vi "L0_SUM_NOISE_TEST.vi"(7 "Serial Number":string="SN_026", 8 "error in (no error)":errorcluster, 11 "Instrument VISA in":T1={"AWG VISA"="AgilentGenerator1", "Oscilloscope  VISA "="AgilentOsciloscope", "Integration Board IP"="172.16.17.47", "connection ID"=refnum, "report out"=refnum, "report file path"=path "C:/Users/omartinez/Desktop/L0nL1_Results"}) -> (0 "error out":errorcluster, 3 "Instrument VISA out":T1={"AWG VISA"="AgilentGenerator1", "Oscilloscope  VISA "="AgilentOsciloscope", "Integration Board IP"="172.16.7.43", "connection ID"=refnum, "report out"=refnum, "report file path"=path "C:/Documents and Settings/CTA_LAB01/Desktop/L0_Asic/L0 Asic Test Data"})   [LabVIEW 2012]
uses:
  <vilib>/Utility/NIReport.llb/NI_report.lvclass
  <vilib>/Utility/NIReport.llb/HTML/NI_HTML.lvclass
  <instrlib>/Agilent 8000 Series/Public/Configure/Configure Math (Binary Operation).vi
  L0&L1/L0_BOARD_TESTs/trunk/Sum_Abrilader/L0_Sum_Adder Folder/C/Program Files/National Instruments/LabVIEW 2012/instr.lib/Agilent 8000 Series/Public/Data/Low Level/Fetch Measurement (More).vi
  <instrlib>/Agilent 8000 Series/Agilent 8000 Series.lvlib
panel:
  in  "Input Voltage":dbl=0.05
  in  "Amp Scaler":dbl=100.0
  in  "Ib_clipVb":u32=63
  in  "Clip_sel_b":u32=1
  in  "Att gain":u32
  in  "Delay value":u16
  in  "Gen Active":bool
  in  "Sum/Maj":bool
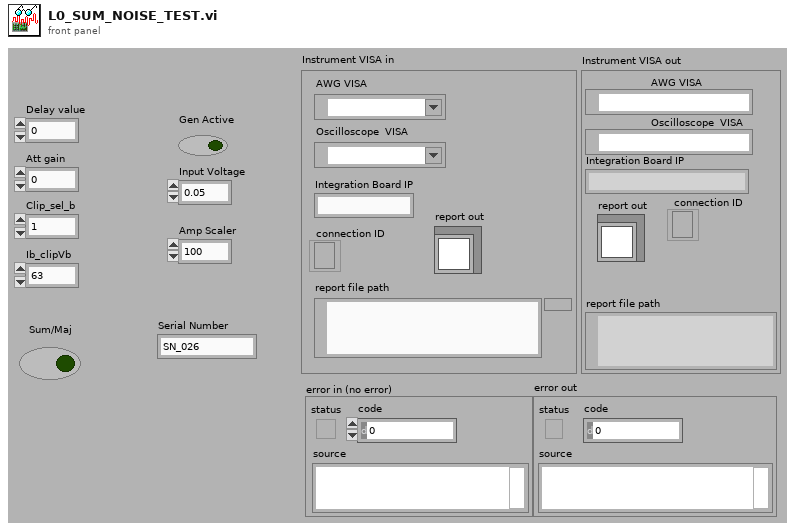
[diagram p1: front panel]
types:
  T1 = cluster{"AWG VISA":refnum<visa-resource-name>, "Oscilloscope  VISA ":refnum<visa-resource-name>, "Integration Board IP":string, "connection ID":refnum<k5>, "report out":refnum<class "NI_report.lvclass">, "report file path":path}
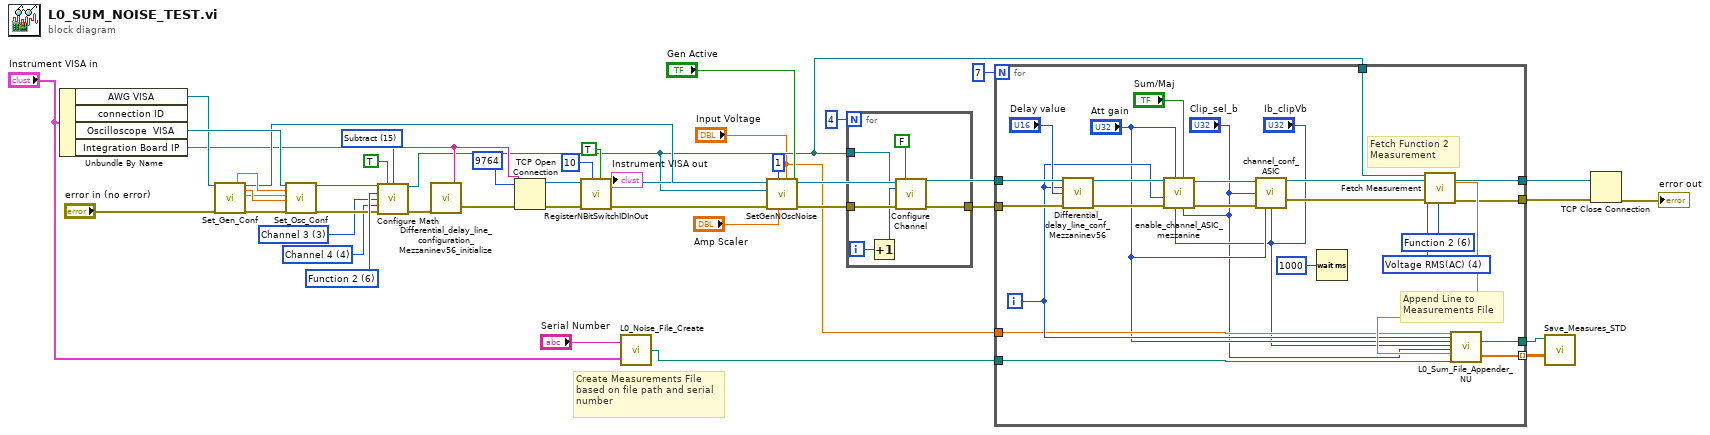
[diagram p0: block diagram]
diagram:
  w20 = u16 6 items=["Function 1"=5, "Function 2"=6, "Function 3"=7, "Function 4"=8] ("Math Channel (5: Function 1)")
  w21 = u16 15 items=["Add"=12, "Divide"=13, "Multiply"=14, "Subtract"=15, "Common Mode"=16, "Versus"=17] ("Math Operation (12: Add)")
  w15 = 3 items=["Channel 1"=1, "Channel 2"=2, "Channel 3"=3, "Channel 4"=4] ("Channel (1: Channel 1)")
  w16 = 4 items=["Channel 1"=1, "Channel 2"=2, "Channel 3"=3, "Channel 4"=4] ("Channel (1: Channel 1)")
  # "Create Measurements File\nbased on file path and serial\nnumber"
  n1 = Unbundle By Name("Instrument VISA in") -> ("AWG VISA"=w38:refnum<visa-resource-name>, "Oscilloscope  VISA"=w39:refnum<visa-resource-name>, "Integration Board IP"=w23:string)  [unwired: 1 out]
  n2 = call "Set_Gen_Conf.vi"("AWG VISA"=w38, "error in (no error)"="error in (no error)") -> ("Amplitude 1 OUT"=w36:dbl, "VISA resource name out"=w29:refnum<visa-resource-name>, "Pulse Width in seconds 1 OUT"=w35:dbl, "Trigger Level 1"=w34:dbl, "error out"=w40:errorcluster)  [unwired: 10 in, 3 out]
  n3 = call "Set_Osc_Conf.vi"("VISA resource name"=w39, "Amplitude IN"=w36, "Trigger Level IN"=w34, "Pulse Width in seconds IN"=w35, "error in (no error)"=w40) -> ("VISA resource name out"=w19:refnum<visa-resource-name>, "error out"=w18:errorcluster)  [unwired: 13 in]
  n4 = call-poly <instrlib>:"Configure Math.vi"("VISA resource name"=w19, "Enable Math Channel (T:Enable)"=TRUE, "Math Operation (12: Add)"=w21, "Math Channel (5: Function 1)"=w20, "Math Operand (1: Channel 1)"=w15, "Math Operand (2: Channel 2)"=w16, "error in (no error)"=w18) -> ("VISA resource name out"=w7:refnum<visa-resource-name>, "error out"=w17:errorcluster)  [unwired: 7 in]
  n5 = call "Differential_delay_line_configuration_Mezzaninev56_initialize.vi"("error in (no error)"=w17, "address"=w23) -> ("error out 2"=w33:errorcluster)
  n6 = TCP Open Connection(address=w23, remote port or service name=9764, error in (no error)=w33) -> (connection ID=w27:refnum<k5>, error out=w32:errorcluster)  [unwired: 2 in]
  n7 = call "RegisterNBitSwitchIDInOut.vi"("Switch Bit"=TRUE, "N Bit"=10, "error in (no error)"=w32, "connection ID"=w27) -> ("error out"=w28:errorcluster, "connection ID out"=w26:refnum<k5>)  [unwired: 5 in]
  n8 = call "L0_Noise_File_Create.vi"("input cluster"="Instrument VISA in", "Serial Number"="Serial Number") -> ("appended path"=w4:path)
  n9 = call "SetGenNOscNoise.vi"("Enable Output"="Gen Active", "Input Voltage"="Input Voltage", "Amp Scaler"="Amp Scaler", "NChannels"=1, "error in (no error)"=w28, "VISA resource name"=w7, "AWG VISA"=w29) -> ("error out 2"=w12:errorcluster)  [unwired: 4 in]
  n10 = for {
    N: 4 -> [_]
    tunnel: w12 -> [w48]
    tunnel: [w47] -> w11
    tunnel: w7 -> [w45]
    i -> [w46]
    n11 = Increment(x=w46) -> (x+1=w43:i32)
    n12 = call <instrlib>:"Configure Channel.vi"("VISA resource name"=w45, "Enable Channel (Enable)"=FALSE, "Channel (1: Channel 1)"=w43, "error in (no error)"=w48) -> ("error out"=w47:errorcluster)  [unwired: 10 in, 1 out]
  }
  n13 = for {
    N: 7 -> [_]
    tunnel: [w58] -> w31
    tunnel: [w72] -> w30
    tunnel: w26 -> [w71]
    tunnel: w11 -> [w63]
    tunnel: w7 -> [w57]
    tunnel: w4 -> [w56]
    tunnel: "Input Voltage" -> [w54]
    tunnel: [w50] -> w2
    tunnel: [w49] -> w1 mode=indexing
    i -> [w55]
    w60 = 4 items=["Rise Time", "Fall Time", "Frequency", "Period", "Voltage RMS(AC)", "Voltage RMS(DC)", "Voltage RMS (AC,cycle)", "Voltage RMS (DC,cycle)", "Voltage Max", "Voltage Min", "Voltage Middle", "Voltage Vpp", "Voltage High", "Voltage Low", "Voltage Average", "Voltage Average (cycle)", "Width Negative", "Width Positive", "Duty Cycle Positive", "Amplitude", "Overshoot", "Preshoot", "Voltage Base", "Voltage Upper", "Time Max", "Time Min", "Color Grade Crossing", "Color Grade Eye Width", "Color Grade Eye Height", "Color Grade Eye Q-Factory", "Color Grade Eye Duty Cycle Distortion(Percent)", "Color Grade Eye Duty Cycle Distortion(Time)", "Color Grade Eye Jitter(PP)", "Color Grade Eye Width(RMS)", "Cycle-cycle Duty Jitter(Rising)", "Cycle-cycle Duty Jitter(Falling)", "Cycle-cycle Jitter(Rising)", "Cycle-cycle Jitter(Falling)", "Cycle-cycle - Width", "Cycle-cycle + Width", "Date Rate", "Unit Interval", "FFT Delta Frequency", "FFT Delta Magnitude", "FFT Frequency", "FFT Magnitude", "Slew Rate", "Area (Entire Display)", "Area(Single Cycle)", "Duty Cycle (Rising)", "Duty Cycle (Falling)"] ("Measurement Function (0: Rise Time)")
    w61 = 6 items=["Channel 1"=1, "Channel 2"=2, "Channel 3"=3, "Channel 4"=4, "Function 1"=5, "Function 2"=6, "Function 3"=7, "Function 4"=8, "Memory 1"=9, "Memory 2"=10, "Memory 3"=11, "Memory 4"=12] ("Channel (1: Channel 1)")
    # "Append Line to \nMeasurements File"
    # "Fetch Function 2\nMeasurement"
    n14 = call "Differential_delay_line_conf_Mezzaninev56.vi"("connection ID"=w71, "channel"=w55, "Delay value"="Delay value", "error in (no error)"=w63) -> ("connection ID out"=w68:refnum<k5>, "error out 2"=w70:errorcluster)  [unwired: 4 in, 6 out]
    n15 = call "enable_channel_ASIC_mezzanine.vi"("Clip_sel_b"="Clip_sel_b", "maj/sum"="Sum/Maj", "Ib_clipVb"="Ib_clipVb", "Att gain"="Att gain", "error in"=w70, "Channel"=w55, "connection ID"=w68) -> ("error out"=w69:errorcluster, "connection ID out"=w67:refnum<k5>)  [unwired: 2 in, 1 out]
    n16 = call "channel_conf_ASIC.vi"("connection ID"=w67, "Clip_sel_b"="Clip_sel_b", "error out"=w69, "Att gain"="Att gain", "Ib_ClipVb"="Ib_clipVb") -> ("connection ID out"=w72:refnum<k5>, "error out 2"=w59:errorcluster)  [unwired: 6 in, 3 out]
    n17 = Wait (ms)(milliseconds to wait=1000) -> ()  [unwired: 1 out]
    n18 = call-poly "Fetch Measurement.vi"("VISA resource name"=w57, "Channel (1: Channel 1)"=w61, "Measurement Function (0: Rise Time)"=w60, "error in (no error)"=w59) -> ("Measurement"=w62:dbl, "error out"=w58:errorcluster)  [unwired: 9 in, 1 out]
    n19 = call "L0_Sum_File_Appender_NU.vi"("Vin"=w54, "CH"=w55, "Att"="Att gain", "IbClip"="Ib_clipVb", "Clip"="Clip_sel_b", "Vmeas"=w62, "file path (dialog if empty)"=w56) -> ("appended array"=w49:dbl[], "file path (dialog if empty) 2"=w50:path)  [unwired: 19 in]
  }
  n20 = call "Save_Measures_STD.vi"("Data in"=w1, "file path (dialog if empty)"=w2) -> ()  [unwired: 10 in]
  n21 = TCP Close Connection(connection ID=w30, error in (no error)=w31) -> (error out=→"error out":errorcluster)  [unwired: 1 in, 1 out]
